vi "getInfo.vi"(0 "GenericMission in":refnum<class "GenericMission.lvclass">, 11 "error in (no error)":errorcluster) -> (1 "Done":bool, 3 "Duration (s)":dbl, 4 "GenericMission out":refnum<class "GenericMission.lvclass">, 6 "Mission Type":T1, 10 "Points of Interest":T2[](array[typedef]) {"North" format="%#_10f"; "East" format="%#_8f"}, 12 "Tolerance (m)":dbl, 13 "Timeout (s)":dbl, 14 "ID#":i16=-1, 15 "error out":errorcluster)   [LabVIEW 2013, in "GenericMission.lvclass"]
doc: "Allows you to access all of the private data of any mission. Should not need to be overridden by child classes."
uses:
  GenericMission.lvclass
  Data/TypeDefs/UTM Location.ctl
  Data/TypeDefs/MissionTypeControl.ctl
  GenericMission.lvclass/GenericMission.ctl
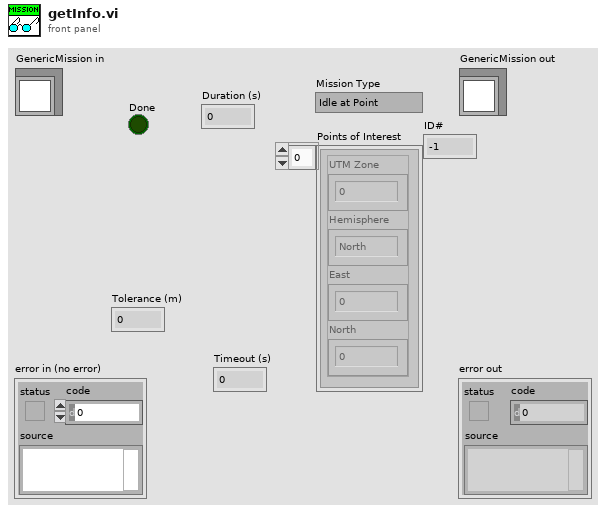
[diagram p1: front panel]
types:
  T1 = typedef "MissionTypeControl.ctl" = enum16{"Idle at Point", "Drive to Waypoint", "Round Buoy to Port", "Round Buoy to Starboard", "Pass Between Buoys", "Station Keeping"}
  T2 = typedef "UTM Location.ctl" = cluster{"UTM Zone":dbl, "Hemisphere":enum16{"North", "South"}, "East":dbl, "North":dbl}
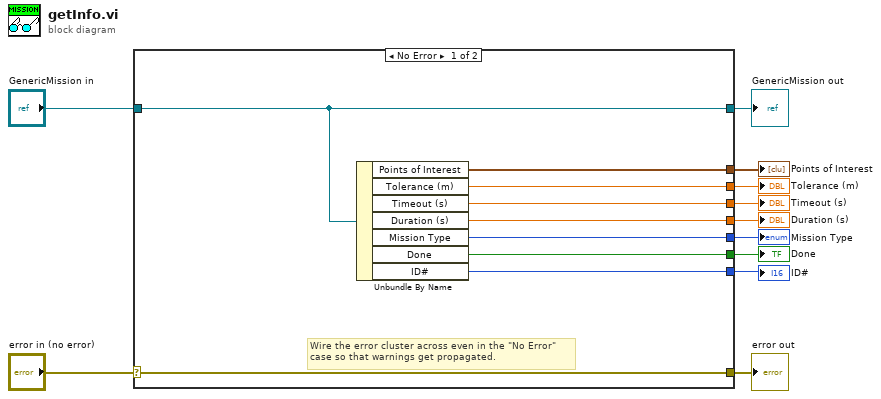
[diagram p0: block diagram]
diagram:
  n1 = case shown="No Error" "error in (no error)" {
    selector: "error in (no error)" -> [w20 w22]
    tunnel: [w20 w22] -> w10
    tunnel: [w19 w21] -> w8
    tunnel: "GenericMission in" -> [w19 w21]
    tunnel: [w18 _] -> w7
    tunnel: [w17 _] -> w6
    tunnel: [w16 _] -> w5
    tunnel: [w15 _] -> w4
    tunnel: [w14 _] -> w3
    tunnel: [w13 _] -> w2
    tunnel: [w12 _] -> w1
    frame No Error {
      # "Wire the error cluster across even in the \"No Error\"\ncase so that warnings get propagated."
      n2 = Unbundle By Name(w19) -> ("Points of Interest"=w18:T2[], "Tolerance (m)"=w17:dbl, "Timeout (s)"=w16:dbl, "Duration (s)"=w15:dbl, "Mission Type"=w14:T1, "Done"=w13:bool, "ID#"=w12:i16)
    }
    frame Error {
    }
  }
  "error out" <- w10
  "GenericMission out" <- w8
  "Points of Interest" <- w7
  "Tolerance (m)" <- w6
  "Timeout (s)" <- w5
  "Duration (s)" <- w4
  "Mission Type" <- w3
  "Done" <- w2
  "ID#" <- w1
